vi "FGen Timer FGV.vi"(7 "Action":T1, 8 "error in (no error)":errorcluster, 10 "Time Target (ms)":dbl format="%#_13g") -> (0 "error out":errorcluster, 1 "Time Elapsed?":bool, 2 "Time Elapsed":dbl)   [LabVIEW 2021]
uses:
  Controls/FGen Timer Enum.ctl
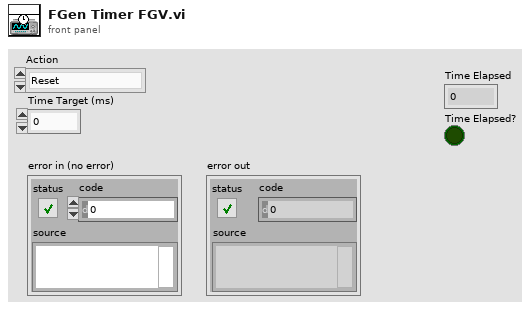
[diagram p1: front panel]
types:
  T1 = typedef "FGen Timer Enum.ctl" = enum16{"Reset", "Time Elapsed", "Set Duration"}
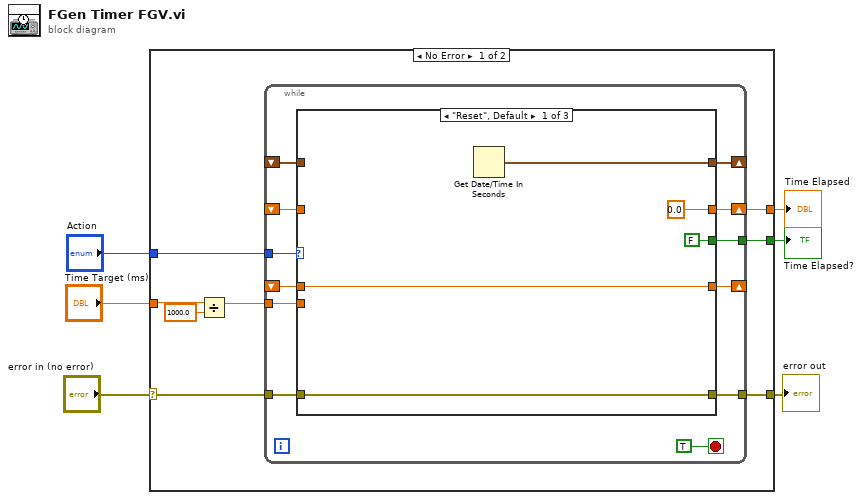
[diagram p0: block diagram]
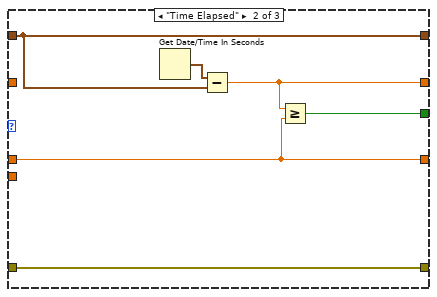
[diagram p2: hidden frame]
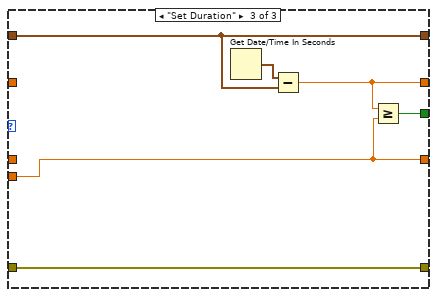
[diagram p3: hidden frame]
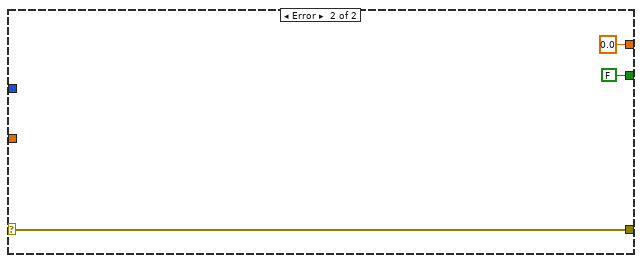
[diagram p4: hidden frame]
diagram:
  n1 = case shown="No Error" "error in (no error)" {
    selector: "error in (no error)" -> [w11 w46]
    tunnel: "Action" -> [w14 _]
    tunnel: "Time Target (ms)" -> [w9 _]
    tunnel: [w13 0.0] -> w4
    tunnel: [w12 FALSE] -> w3
    tunnel: [w10 w46] -> w1
    frame No Error {
      n2 = Divide(x=w9, y=1000.0) -> (x/y=w7:dbl)
      n3 = while {
        tunnel: w14 -> [w25]
        shift-right: [w24] -> _
        shift-left: _ -> [w23]
        shift-right: [w22] -> w13
        shift-left: _ -> [w21]
        tunnel: w7 -> [w20]
        shift-right: [w19] -> _
        shift-left: _ -> [w18]
        tunnel: [w17] -> w12
        tunnel: w11 -> [w16]
        tunnel: [w15] -> w10
        stop <- TRUE stop-if-true
        n4 = case shown="\"Reset\", Default" w25 {
          tunnel: [w31 w36 w40] -> w24
          tunnel: w23 -> [_ w36 w40]
          tunnel: [0.0 w35 w39] -> w22
          tunnel: w21 -> [_ _ _]
          tunnel: w20 -> [_ _ w43]
          tunnel: [w27 w34 w43] -> w19
          tunnel: w18 -> [w27 w34 _]
          tunnel: [FALSE w33 w42] -> w17
          tunnel: w16 -> [w28 w32 w38]
          tunnel: [w28 w32 w38] -> w15
          frame "Reset", Default {
            n5 = Get Date/Time In Seconds() -> (seconds since 1Jan1904=w31:timestamp)
          }
          frame "Time Elapsed" {
            n6 = Get Date/Time In Seconds() -> (seconds since 1Jan1904=w37:timestamp)
            n7 = Subtract(x=w37, y=w36) -> (x-y=w35:dbl)
            n8 = Greater Or Equal?(x=w35, y=w34) -> (x >= y?=w33:bool)
          }
          frame "Set Duration" {
            n9 = Get Date/Time In Seconds() -> (seconds since 1Jan1904=w41:timestamp)
            n10 = Subtract(x=w41, y=w40) -> (x-y=w39:dbl)
            n11 = Greater Or Equal?(x=w39, y=w43) -> (x >= y?=w42:bool)
          }
        }
      }
    }
    frame Error {
    }
  }
  "Time Elapsed" <- w4
  "Time Elapsed?" <- w3
  "error out" <- w1
